vi "ClientSDO_writeByteArray.vi"(6 "Value in":u8[](array[numeric]), 8 "error in (no error)":errorcluster, 9 "sub_index":u8, 10 "object_index":u16 format="%.0x", 11 "ClientSDO Ref in":refnum<k24>) -> (0 "error IO":errorcluster, 1 "ErrorCode":u32, 2 "status":i32(ring) items=["CANOPEN_OK"=0, "CANOPEN_ERROR"=-255, "CANOPEN_ERROR_ASYNC_TRANSFER_ENABLED"=-114, "CANOPEN_ASYNC_TRANSFER"=-113, "CANOPEN_ERROR_NOT_EDS_DCF_CONFIGURED"=-112, "CANOPEN_ERROR_FILE_NOT_FOUND"=-111, "CANOPEN_ERROR_NOT_IMPLEMENTED"=-110, "CANOPEN_ERROR_NO_MESSAGE"=-109, "CANOPEN_UNSUPPORTED_BITRATE"=-108, "CANOPEN_OUT_OF_CAN_INTERFACES"=-107, "CANOPEN_ERROR_DRIVER"=-106, "CANOPEN_ERROR_HW_UNDEFINED"=-105, "CANOPEN_ERROR_HW_NOT_CONNECTED"=-104, "CANOPEN_ERROR_HW_CONNECTED"=-103, "CANOPEN_ERROR_CAN_LAYER_OVRFLOW"=-102, "CANOPEN_ERROR_CAN_LAYER"=-101, "CANOPEN_CAN_LAYER_FAILED"=-100, "CANOPEN_NODE_ID_OUT_OF_RANGE"=-15, "CANOPEN_INTERNAL_STATE_ERROR"=-14, "CANOPEN_CMD_SPEC_UNKNOWN_OR_INVALLD"=-13, "CANOPEN_ERR_DEFINED_BY_APPL"=-12, "CANOPEN_OUT_OF_MEM"=-11, "CANOPEN_REMOTE_NODE_ABORT"=-10, "CANOPEN_APP_BUF_OUT_OF_RANGE"=-9, "CANOPEN_OBJECT_MISSMATCH"=-8, "CANOPEN_BUFFER_TOO_SMALL"=-7, "CANOPEN_TOGGLE"=-6, "CANOPEN_MSG_NOT_PROCESSED"=-5, "CANOPEN_TIMEOUT"=-4, "CANOPEN_UNEXPECTED_CCS"=-3, "CANOPEN_UNEXPECTED_SCS"=-2, "CANOPEN_ARG_ERROR"=-1], 3 "ClientSDO Ref out":refnum<k24>)   [LabVIEW 2015, in "CANOpen.lvlib"]
doc: "write an array of byte to <b>client</b> using SDO protocol"
uses:
  CANOpen.lvlib
  \\Mac\Home/Desktop/imt_test_app 28-06-2012/canopenlib_cli.dll
  canopenlib_cli.dll
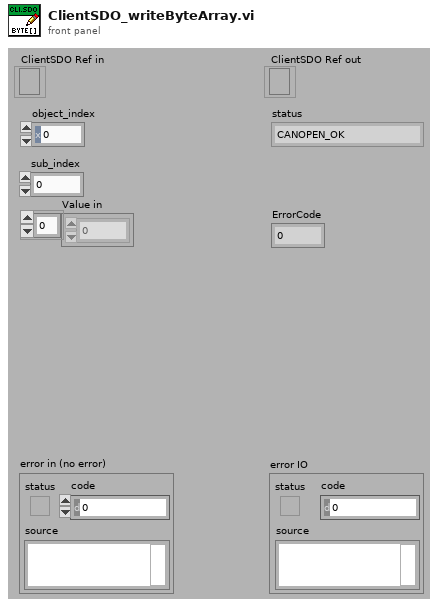
[diagram p1: front panel]
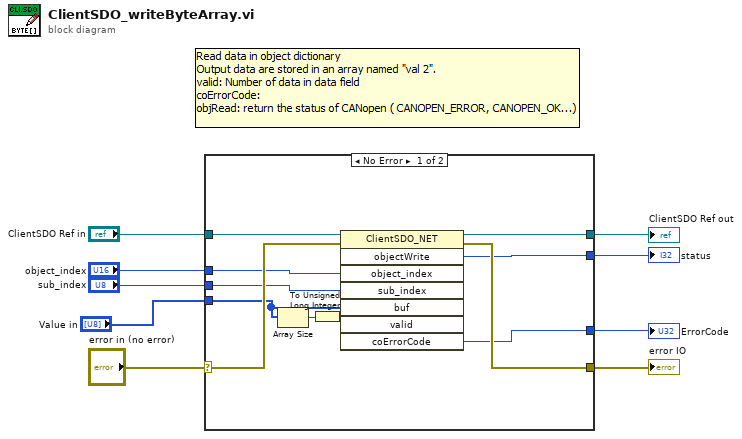
[diagram p0: block diagram]
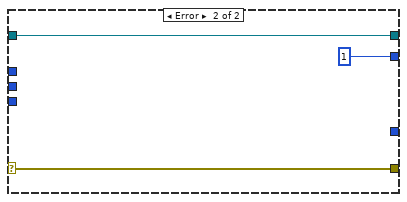
[diagram p2: hidden frame]
diagram:
  n1 = case shown="No Error" "error in (no error)" {
    selector: "error in (no error)" -> [w19 w22]
    tunnel: "ClientSDO Ref in" -> [w20 w23]
    tunnel: "object_index" -> [w18 _]
    tunnel: "sub_index" -> [w17 _]
    tunnel: [w16 w23] -> w5
    tunnel: [w15 w22] -> w4
    tunnel: [w14 1 ("objectRead")] -> w1
    tunnel: [w13 _] -> w2
    tunnel: "Value in" -> [w11 _]
    frame No Error {
      n2 = Array Size(array=w11) -> (size(s)=w12:i32)
      n3 = To Unsigned Long Integer(number=w12) -> (unsigned 32bit integer=w10:u32)
      n4 = invoke class="ClientSDO_NET" method="objectWrite"(reference=w20, error in=w19, "object_index"=w18, "sub_index"=w17, "buf"=w11, "valid"=w10) -> (reference out=w16:refnum<k24>, error out=w15:errorcluster, "objectWrite"=w14:i32, "coErrorCode"=w13:u32)  [unwired: 2 in, 4 out]
    }
    frame Error {
    }
  }
  "ClientSDO Ref out" <- w5
  "error IO" <- w4
  "ErrorCode" <- w2
  "status" <- w1
